vi "Auto Baller Turn.vi"(9 "Right Drive":dbl, 10 "Left Drive":dbl, 11 "Run?":bool) -> (3 "Done":bool)   [LabVIEW 2013]
panel:
  out "Left":dbl
  out "Right":dbl
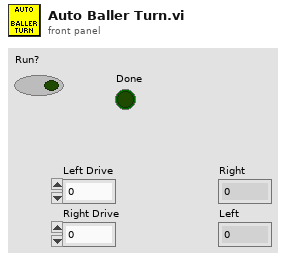
[diagram p1: front panel]
types:
  T1 = typedef "WPI_EncoderDevRef.ctl" = cluster{"DevStatus":errorcluster, "EncoderIndex":T2, "CounterIndex":T3, "DistancePerCount":dbl, "Decoding Type":T4}
  T2 = typedef "FPGA_EncoderIdx.ctl" = enum8{"Enc 0", "Enc 1", "Enc 2", "Enc 3", "Invalid"}
  T3 = typedef "FPGA_CounterCtrSystemIndex.ctl" = enum8{"Ctr 0", "Ctr 1", "Ctr 2", "Ctr 3", "Ctr 4", "Ctr 5", "Ctr 6", "Ctr 7", "Invalid"}
  T4 = typedef "WPI_EncoderType.ctl" = enum16{"1x", "2x", "4x"}
  T5 = typedef "WPI_MotorControlDeviceRef.ctl" = cluster{"DeviceStatus":errorcluster, "Type":enum16{"PWM", "CAN"}, "PWM":cluster{"Digital Module":T6, "PWM Channel":T7, "DeadBand":T8}, "CAN":cluster{"Device Number":u8, "Control Mode":T9, "Semaphore":T10, "Max Vout":dbl}, "Invert":bool, "TransformRef":T11, "InvTransformRef":T11}
  T6 = typedef "FPGA_TypedefDigitalModule.ctl" = enum16{"Digital Module 1", "Digital Module 2"}
  T7 = typedef "FPGA_DIOPWMChannel.ctl" = enum8{"PWM 1", "PWM 2", "PWM 3", "PWM 4", "PWM 5", "PWM 6", "PWM 7", "PWM 8", "PWM 9", "PWM 10", "Invalid"}
  T8 = typedef "WPI_PWMDeadband.ctl" = cluster{"Name":string, "maxPositivePwm":i32, "minPositivePwm":i32, "centerPwm":i32, "maxNegativePwm":i32, "minNegativePwm":i32, "angularRange":u16}
  T9 = typedef "WPI_CANJaguar_ControlMode.ctl" = enum8{"Percent VBus", "Current", "Speed", "Position", "Voltage"}
  T10 = typedef "Semaphore RefNum" = refnum<k1>
  T11 = typedef "WPI_PWMTransform_ConPane.ctl" = refnum<vi>
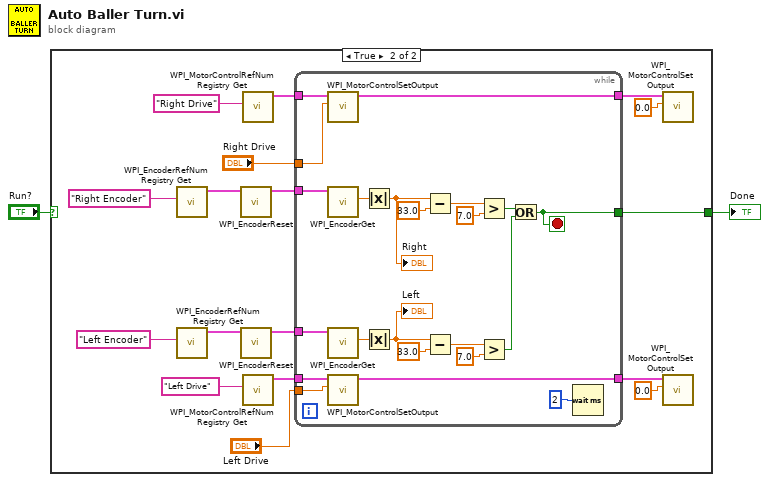
[diagram p0: block diagram]
diagram:
  n1 = case shown="True" "Run?" {
    selector: "Run?" -> [w3 _]
    tunnel: [w3 w8] -> w1
    frame False {
    }
    frame True {
      n2 = call <vilib>:"WPI_EncoderRefNum Registry Get.vi"("refnum name"="Right Encoder") -> ("EncoderDevRef"=w10:T1)  [unwired: 9 in, 1 out]
      n3 = call <vilib>:"WPI_EncoderRefNum Registry Get.vi"("refnum name"="Left Encoder") -> ("EncoderDevRef"=w14:T1)  [unwired: 9 in, 1 out]
      n4 = call <vilib>:"WPI_EncoderReset.vi"("EncoderDevRef"=w10) -> ("EncoderDevRef"=w9:T1)  [unwired: 9 in, 1 out]
      n5 = call <vilib>:"WPI_EncoderReset.vi"("EncoderDevRef"=w14) -> ("EncoderDevRef"=w12:T1)  [unwired: 9 in, 1 out]
      n6 = call <vilib>:"WPI_MotorControlRefNum Registry Get.vi"("refnum name"="Right Drive") -> ("MotorControlDevRef"=w17:T5)  [unwired: 9 in, 1 out]
      n7 = call <vilib>:"WPI_MotorControlRefNum Registry Get.vi"("refnum name"="Left Drive") -> ("MotorControlDevRef"=w20:T5)  [unwired: 9 in, 1 out]
      n8 = while {
        tunnel: w20 -> [w40]
        tunnel: w17 -> [w39]
        tunnel: "Left Drive" -> [w38]
        tunnel: "Right Drive" -> [w37]
        tunnel: w12 -> [w36]
        tunnel: w9 -> [w25]
        tunnel: [w23] -> w8
        tunnel: [w22] -> w7
        tunnel: [w21] -> w5
        stop <- w23 stop-if-true
        n9 = call <vilib>:"WPI_MotorControlSetOutput.vi"("Output"=w37, "MotorControlDevRef"=w39) -> ("MotorControlDevRef"=w21:T5)  [unwired: 7 in, 2 out]
        n10 = call <vilib>:"WPI_EncoderGet.vi"("EncoderDevRef"=w25) -> ("Distance"=w24:dbl)  [unwired: 5 in, 5 out]
        n11 = call <vilib>:"WPI_EncoderGet.vi"("EncoderDevRef"=w36) -> ("Distance"=w26:dbl)  [unwired: 5 in, 5 out]
        n12 = call <vilib>:"WPI_MotorControlSetOutput.vi"("Output"=w38, "MotorControlDevRef"=w40) -> ("MotorControlDevRef"=w22:T5)  [unwired: 7 in, 2 out]
        n13 = Absolute Value(x=w24) -> (abs(x)=w28:dbl)
        "Right" <- w28
        n14 = Absolute Value(x=w26) -> (abs(x)=w27:dbl)
        "Left" <- w27
        n15 = Subtract(x=w28, y=33.0) -> (x-y=w31:dbl)
        n16 = Subtract(x=w27, y=33.0) -> (x-y=w32:dbl)
        n17 = Greater?(x=w31, y=7.0) -> (0:w33:bool)
        n18 = Greater?(x=w32, y=7.0) -> (0:w35:bool)
        n19 = Or(x=w33, y=w35) -> (x .or. y?=w23:bool)
        n20 = Wait (ms)(milliseconds to wait=u32 2) -> ()  [unwired: 1 out]
      }
      n21 = call <vilib>:"WPI_MotorControlSetOutput.vi"("Output"=0.0, "MotorControlDevRef"=w5) -> ()  [unwired: 7 in, 3 out]
      n22 = call <vilib>:"WPI_MotorControlSetOutput.vi"("Output"=0.0, "MotorControlDevRef"=w7) -> ()  [unwired: 7 in, 3 out]
    }
  }
  "Done" <- w1
